vi "限幅器（TimeStamp[]）.vi"(3 "下限":timestamp, 4 "X_in":timestamp[](array[timestamp]), 5 "上限":timestamp) -> (1 "X_Out":timestamp[](array[timestamp]))   [LabVIEW 2012]
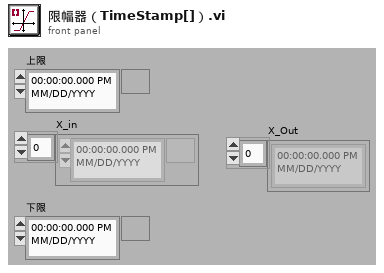
[diagram p1: front panel]
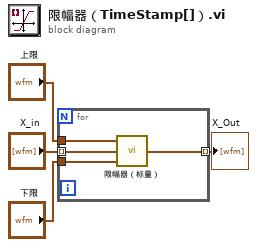
[diagram p0: block diagram]
diagram:
  n1 = for {
    tunnel: "X_in" -> [w8] mode=indexing
    tunnel: "上限" -> [w7]
    tunnel: "下限" -> [w6]
    tunnel: [w5] -> w1 mode=indexing
    n2 = call-poly "限幅器（标量）.vi"("下限"=w6, "X_in"=w8, "上限"=w7) -> ("X_Out"=w5:timestamp)  [unwired: 2 in]
  }
  "X_Out" <- w1
